vi "Write Error.vi"(8 "error in (no error)":errorcluster, 11 "Error String":string) -> (0 "error out":errorcluster, 2 "Valid File?":bool, 3 "Error_Log":path)   [LabVIEW 2024]
uses:
  Variables/Download Confrigurations.vi
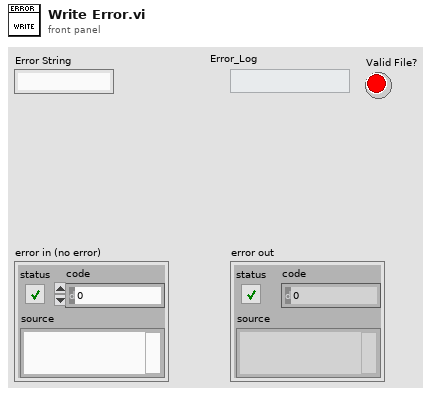
[diagram p1: front panel]
types:
  T1 = enum16{"open", "replace", "create", "open or create", "replace or create", "replace or create with confirmation"}
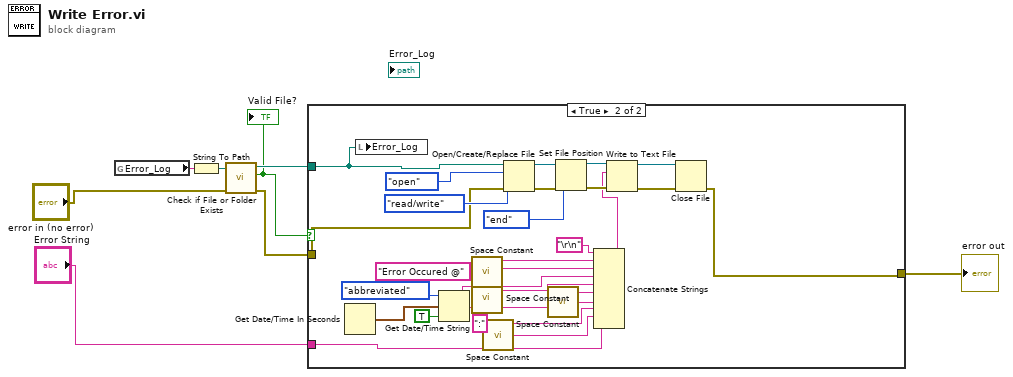
[diagram p0: block diagram]
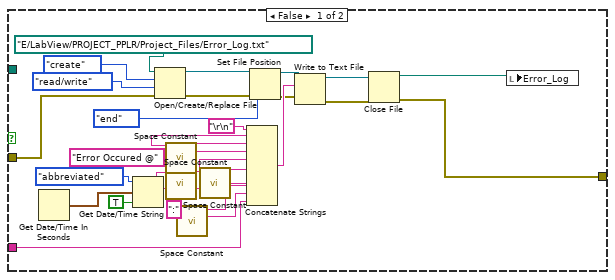
[diagram p2: hidden frame]
diagram:
  n1 = global read "Download Confrigurations.vi" "Error_Log"() -> (w1:string)
  n2 = String To Path(string=w1) -> (path=w2:path)
  n3 = call <vilib>:"Check if File or Folder Exists.vi"("error in (no error)"="error in (no error)", "path"=w2) -> ("error out"=w6:errorcluster, "file or folder exists?"=w4:bool, "dup path"=w5:path)  [unwired: 7 in]
  "Valid File?" <- w4
  n4 = case shown="True" w4 {
    tunnel: w5 -> [_ w44]
    tunnel: w6 -> [w32 w59]
    tunnel: "Error String" -> [w19 w47]
    tunnel: [w18 w51] -> w8
    frame False {
      n5 = Get Date/Time In Seconds() -> (seconds since 1Jan1904=w25:timestamp)
      n6 = Get Date/Time String(date format (0)=enum16{"short", "long", "abbreviated"}."abbreviated", seconds (now)=w25, want seconds? (F)=TRUE) -> (date string=w27:string, time string=w29:string)
      n7 = Open/Create/Replace File(file path (use dialog)=path "E:/LabView/PROJECT_PPLR/Project_Files/Error_Log.txt", error in=w32, operation (0:open)=T1."create", access (0:read/write)=enum16{"read/write", "read-only", "write-only"}."read/write") -> (refnum out=w10:refnum<file>, error out=w9:errorcluster)  [unwired: 2 in, 1 out]
      n8 = call <vilib>:"Space Constant.vi"() -> ("String"=w26:string)
      n9 = call <vilib>:"Space Constant.vi"() -> ("String"=w28:string)
      n10 = call <vilib>:"Space Constant.vi"() -> ("String"=w31:string)
      n11 = call <vilib>:"Space Constant.vi"() -> ("String"=w30:string)
      n12 = Concatenate Strings("\r\n", "Error Occured @" ("string"), w26, w27, w28, w29, w30, ":", w31, w19) -> (w15:string)
      n13 = Set File Position(refnum=w10, from (0:start)=enum16{"start", "end", "current"}."end", error in=w9) -> (refnum out=w16:refnum<file>, error out=w14:errorcluster)  [unwired: 1 in]
      n14 = Write to Text File(file (use dialog)=w16, text=w15, error in=w14) -> (refnum out=w13:refnum<file>, error out=w12:errorcluster)  [unwired: 1 in, 1 out]
      n15 = Close File(refnum=w13, error in=w12) -> (path=w11:path, error out=w18:errorcluster)
      n16 = local write "Error_Log"(w11) -> ()
    }
    frame True {
      n17 = Get Date/Time In Seconds() -> (seconds since 1Jan1904=w57:timestamp)
      n18 = local write "Error_Log"(w44) -> ()
      n19 = Get Date/Time String(date format (0)=enum16{"short", "long", "abbreviated"}."abbreviated", seconds (now)=w57, want seconds? (F)=TRUE) -> (date string=w54:string, time string=w52:string)
      n20 = call <vilib>:"Space Constant.vi"() -> ("String"=w55:string)
      n21 = call <vilib>:"Space Constant.vi"() -> ("String"=w53:string)
      n22 = call <vilib>:"Space Constant.vi"() -> ("String"=w48:string)
      n23 = Open/Create/Replace File(file path (use dialog)=w44, error in=w59, operation (0:open)=T1."open", access (0:read/write)=enum16{"read/write", "read-only", "write-only"}."read/write") -> (refnum out=w42:refnum<file>, error out=w43:errorcluster)  [unwired: 2 in, 1 out]
      n24 = call <vilib>:"Space Constant.vi"() -> ("String"=w50:string)
      n25 = Set File Position(refnum=w42, from (0:start)=enum16{"start", "end", "current"}."end", error in=w43) -> (refnum out=w39:refnum<file>, error out=w40:errorcluster)  [unwired: 1 in]
      n26 = Concatenate Strings("\r\n", "Error Occured @" ("string"), w55, w54, w53, w52, w50, ":", w48, w47) -> (w38:string)
      n27 = Write to Text File(file (use dialog)=w39, text=w38, error in=w40) -> (refnum out=w37:refnum<file>, error out=w36:errorcluster)  [unwired: 1 in, 1 out]
      n28 = Close File(refnum=w37, error in=w36) -> (error out=w51:errorcluster)  [unwired: 1 out]
    }
  }
  "error out" <- w8
